vi "Variant_to_Enum_U64.vi"(8 "Error in":errorcluster, 11 "Value (in)":variant) -> (0 "Error out":errorcluster, 2 "Value (string)":string, 3 "Value (out)":u64(ring) items=["fbfgb", "gbfgb", "rtt"])   [LabVIEW 2012]
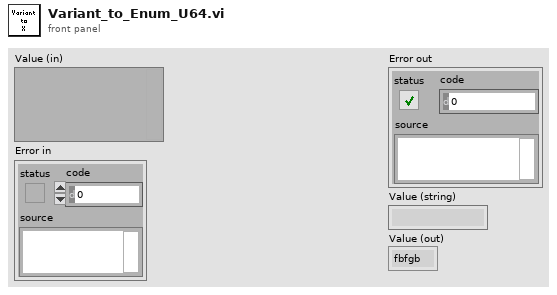
[diagram p1: front panel]
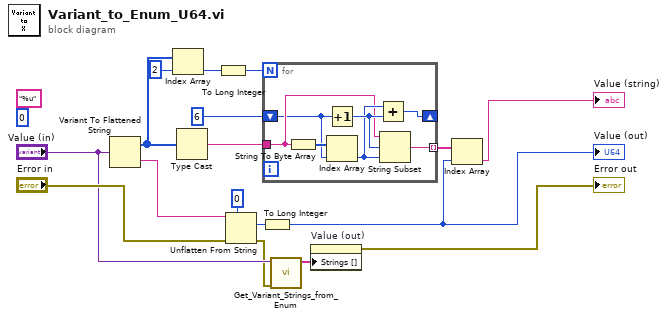
[diagram p0: block diagram]
diagram:
  (unwired) "%u" ("format string")
  (unwired) u16 0
  n1 = Variant To Flattened String(Variant="Value (in)") -> (data string=w12:string, 1:w16:i16[])
  n2 = Index Array(array=w16, index=2) -> (element=w7:i16)
  n3 = Type Cast(x=w16) -> (*(type *) &x=w13:string)  [unwired: 1 in]
  n4 = To Long Integer(number=w7) -> (32bit integer=w6:i32)
  n5 = Unflatten From String(type=u64 0, binary string=w12, error in (no error)="Error in") -> (value=w8:u64, error out=w2:errorcluster)  [unwired: 2 in, 1 out]
  n6 = To Long Integer(number=w8) -> (32bit integer=w5:i32)
  "Value (out)" <- w5
  n7 = for {
    N: w6 -> [_]
    tunnel: w13 -> [w21]
    shift-right: [w20] -> _
    shift-left: 6 ("index") -> [w18]
    tunnel: [w19] -> w15 mode=indexing
    n8 = String To Byte Array(string=w21) -> (unsigned byte array=w24:u8[])
    n9 = Increment(x=w18) -> (x+1=w23:i32)
    n10 = Index Array(array=w24, index=w18) -> (element=w22:u8)
    n11 = Add(x=w22, y=w23) -> (x+y=w20:i32)
    n12 = String Subset(string=w21, offset (0)=w23, length (rest)=w22) -> (substring=w19:string)
  }
  n13 = call "Get_Variant_Strings_from_Enum.vi"("error in (no error)"=w2, "Enum"="Value (in)") -> ("Enum strings"=w1:string[])  [unwired: 6 in, 3 out]
  n14 = property on="Value (out)" class="Ring (strict)"("Strings []"=w1) -> (error out=→"Error out":errorcluster)  [unwired: 2 in, 1 out]
  n15 = Index Array(array=w15, index=w5) -> (element=→"Value (string)":string)
